vi "close.vi"(8 "error in (no error)":errorcluster, 11 "file descriptor in":i32) -> (0 "error out":errorcluster)   [LabVIEW 2013, in "Linux RT IPC.lvlib" / "Pipes.lvlib"]
uses:
  Pipes.lvlib
  Controls/functions.ctl
  <vilib>/NI/NI Linux RT Errno/Linux Errno.lvlib
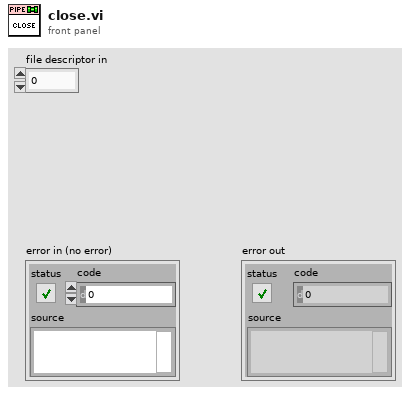
[diagram p1: front panel]
types:
  T1 = typedef "Linux RT IPC.lvlib/Pipes.lvlib/functions.ctl" = enum16{"unspecified", "mkfifo", "open", "read", "write", "close", "unlink"}
  T2 = typedef "Linux Errno.lvlib/errno.ctl" = enum16{"NO ERROR", "EPERM", "ENOENT", "ESRCH", "EINTR", "EIO", "ENXIO", "E2BIG", "ENOEXEC", "EBADF", "ECHILD", "EAGAIN", "ENOMEM", "EACCES", "EFAULT", "ENOTBLK", "EBUSY", "EEXIST", "EXDEV", "ENODEV", "ENOTDIR", "EISDIR", "EINVAL", "ENFILE", "EMFILE", "ENOTTY", "ETXTBSY", "EFBIG", "ENOSPC", "ESPIPE", "EROFS", "EMLINK", "EPIPE", "EDOM", "ERANGE", "EDADLK", "ENAMETOOLONG", "ENOLCK", "ENOSYS", "ENOTEMPTY", "ELOOP", "EWOULDBLOCK", "ENOMSG", "EIDRM", "ECHRNG", "EL2NSYNC", "EL3HLT", "EL3RST", "ELNRNG", "EUNATCH", "ENOCSI", "EL2HLT", "EBADE", "EBADR", "EXFULL", "ENOANO", "EBADRQC", "EBADSLT", "EDEADLOCK", "EBFONT", "ENOSTR", "ENODATA", "ETIME", "ENOSR", "ENONET", "ENOPKG", "EREMOTE", "ENOLINK", "EADV", "ESRMNT", "ECOMM", "EPROTO", "EMULTIHOP", "EDOTDOT", "EBADMSG", "EOVERFLOW", "ENOTUNIQ", "EBADFD", "EREMCHG", "ELIBACC", "ELIBBAD", "ELIBSCN", "ELIBMAX", "ELIBEXEC", "ELISEQ", "ERESTART", "ESTRPIPE", "EUSERS", "ENOTSOCK", "EDESTADDRREQ", "EMSGSIZE", "EPROTOTYPE", "ENOPROTOOPT", "EPROTONOSUPPORT", "ESOCKTNOSUPPORT", "EOPNOTSUPP", "EPFNOSUPPORT", "EAFNOSUPPORT", "EADDRINUSE", "EADDRNOTAVAIL", "ENETDOWN", "ENETUNREACH", "ENETRESET", "ECONNABORTED", "ECONNRESET", "ENOBUFS", "EISCONN", "ENOTCONN", "ESHUTDOWN", "ETOOMANYREFS", "ETIMEDOUT", "ECONNREFUSED", "EHOSTDOWN", "EHOSTUNREACH", "EALREADY", "EINPROGRESS", "ESTALE", "EUCLEAN", "ENOTNAM", "ENAVAIL", "EISNAM", "EREMOTEIO", "EDQUOT", "ENOMEDIUM", "EMEDIUMTYPE", "ECANCELED", "ENOKEY", "EKEYEXPIRED", "EKEYREVOKED", "EKEYREJECTED", "EOWNERDEAD", "ENOTRECOVERABLE", "ERFKILL", "EHWPOISON", "UNDEFINED"}
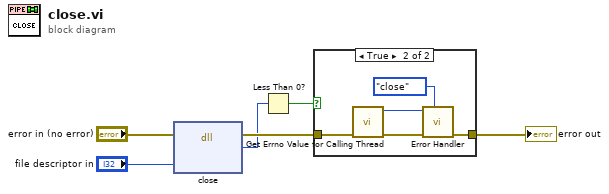
[diagram p0: block diagram]
diagram:
  n1 = dll-call lib="LabVIEW" fn="close"(error in="error in (no error)", "fd"="file descriptor in") -> (error out=w4:errorcluster, "return"=w1:i32)  [unwired: 3 in, 1 out]
  n2 = Less Than 0?(x=w1) -> (x < 0?=w2:bool)
  n3 = case shown="True" w2 {
    tunnel: w4 -> [w7 w12]
    tunnel: [w7 w11] -> w3
    frame False {
    }
    frame True {
      n4 = call <vilib>:"Get Errno Value for Calling Thread.vi"("error in (no error)"=w12) -> ("error out"=w9:errorcluster, "errno"=w10:T2)  [unwired: 9 in]
      n5 = call "Error Handler.vi"("function (unspecified)"=functions."close", "error in (no error)"=w9, "errno"=w10) -> ("error out"=w11:errorcluster)  [unwired: 8 in]
    }
  }
  "error out" <- w3
